vi "close.vi"(8 "error in (no error)":errorcluster, 11 "Pistofono in":refnum<class "Pistofono.lvclass">) -> (0 "error out":errorcluster, 3 "Pistofono out":refnum<class "Pistofono.lvclass">)   [LabVIEW 2019, in "Pistofono.lvclass"]
uses:
  Pistofono.lvclass
  Pistofono.lvclass/Pistofono.ctl
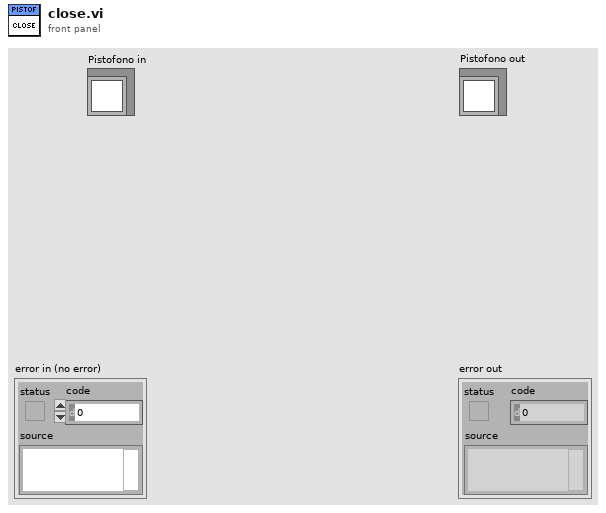
[diagram p1: front panel]
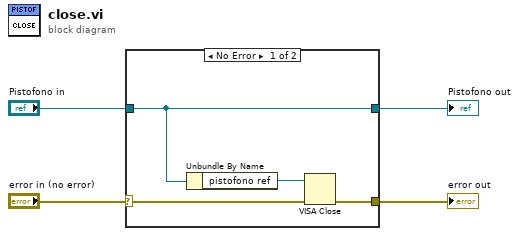
[diagram p0: block diagram]
diagram:
  n1 = case shown="No Error" "error in (no error)" {
    selector: "error in (no error)" -> [w8 w10]
    tunnel: [w7 w10] -> w3
    tunnel: [w6 w9] -> w1
    tunnel: "Pistofono in" -> [w6 w9]
    frame No Error {
      n2 = Unbundle By Name(w6) -> ("pistofono ref"=w5:refnum<visa-resource-name>)
      n3 = VISA Close(VISA resource name=w5, error in (no error)=w8) -> (error out=w7:errorcluster)
    }
    frame Error {
    }
  }
  "error out" <- w3
  "Pistofono out" <- w1
